vi "GUILoop_plotUpdate_cmds.vi"(0 "reference":refnum<class "OSA.lvclass">, 2 "action data in":T1[](array[typedef]) {"par 4" format="%.2f"; "par 3" format="%.2f"; "par 2" format="%.2f"; "par" format="%.2f"}, 5 "error in (no error)":errorcluster, 6 "action interferogram":cluster{"action":T2, "skip old":bool}[](array[cluster]), 8 "action spectrum":cluster{"action":T2, "skip old":bool}[](array[cluster])) -> (14 "reference out":refnum<class "OSA.lvclass">, 16 "action data out":T1[](array[typedef]) {"par 4" format="%.2f"; "par 3" format="%.2f"; "par 2" format="%.2f"; "par" format="%.2f"}, 19 "error out":errorcluster)   [LabVIEW 2010, in "OSA.lvclass"]
doc: "SubVI to a <B>Thorlabs_OSA_64</B> object.\n\n[GOOP 1.0]"
uses:
  OSA.lvclass
  typeDef/queue_action.ctl
  action_data.ctl
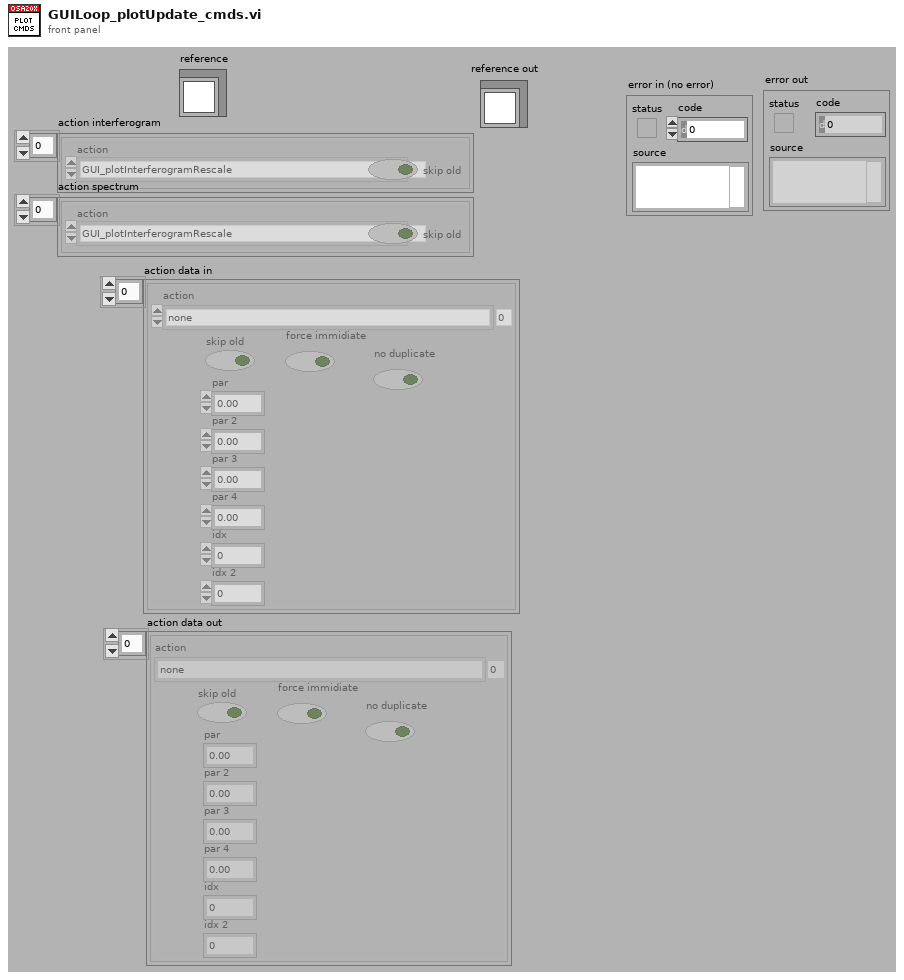
[diagram p1: front panel]
types:
  T1 = typedef "OSA.lvclass/action_data.ctl" = cluster{"action":T2, "skip old":bool, "force immidiate":bool, "par":dbl, "par 2":dbl, "par 3":dbl, "par 4":dbl, "idx":i32, "idx 2":i32, "no duplicate":bool}
  T2 = typedef "OSA.lvclass/queue_action.ctl" = enum16{"none", "stop", "GUI_plotInterferogram", "GUI_plotSpectrum", "GUI_plotInterferogramRescale", "GUI_plotSpectrumRescale", "GUI_plotInterferogramReset", "GUI_plotSpectrumReset", "GUI_plotInterferogramAutoScaleY", "GUI_plotSpectrumAutoScaleY", "GUI_plotInterferogramZoomOut", "GUI_plotSpectrumZoomOut", "GUI_plotInterferogramPane", "GUI_plotSpectrumPane", "GUI_plotInterferogramZoomMouse", "GUI_plotSpectrumZoomMouse", "GUI_plotSpectrumFSRY", "GUI_plotInterferogramFSRY", "GUI_spectrumChannelType", "GUI_channel", "ENVIRONMENT temperature", "ENVIRONMENT pressure", "MODE_resolution set", "MODE_resolution get", "MODE_sensitivity set", "MODE_sensitivity get", "MODE_PDTemperature set", "MODE_PDTemperature get", "REBOOT/RESET firmware", "ACQASYNC_acquireSingleSpectrum", "ACQASYNC_continuous start", "ACQASYNC_continuous stop\n", "ACQASYNC_get last interferogram", "ACQASYNC_get last spectrum", "ACQASYNC_get last waveNr", "ACQOPT_interferogram smoothing set", "ACQOPT_interferogram smoothing get", "ACQOPT_spectrum smoothing set", "ACQOPT_spectrum smoothing get", "ACQOPT_apodisation type set", "ACQOPT_apodisation type get", "ACQOPT_phase correction type set", "ACQOPT_phase correction type get", "ACQOPT_acqIntervall_set", "ACQOPT_acqIntervall_get", "ACQOPT_average spectrum set", "ACQOPT_average spectrum get", "ACQOPT_rolling average set", "ACQOPT_rolling average get", "ACQOPT_zero fill factor set", "ACQOPT_zero fill factor get", "ACQOPT_cycle counting set", "ACQOPT_cycle counting get", "ACQOPT_air measure option set", "ACQOPT_air measure option get", "ACQOPT_gainLevel auto get", "ACQOPT_gainLevel auto set", "ACQOPT_gainLevel get", "ACQOPT_gainLevel set", "ACQOPT_offset set", "ACQOPT_attenuator_auto_set", "ACQOPT_attenuator_set", "ACQOPT_getAll", "INSTRUMENT_PROPERTY_range_WaveNr_min", "INSTRUMENT_PROPERTY_range_WaveNr_max", "INSTRUMENT_PROPERTY_reference_wavelength_cm^-1", "INSTRUMENT_PROPERTY_samplesPerRefPeriod", "INSTRUMENT_PROPERTY_resolution_waveNrPercm", "INSTRUMENT_PROPERTY_availableGainLevels", "INSTRUMENT_PROPERTY_status", "CONVERT", "ANALYSE_POWER", "ANALYSE_PEAKS", "ANALYSE_WAVELENGTH", "ANALYSE_SPECTRUM", "ANALYSE_INTERFEROGRAM", "ANALYSE_COHERENCE_LENGTH", "MATH", "MATH_power", "MATH_peaks", "FILE", "miscellaneous"}
  T3 = typedef "OSA.lvclass/acq_dataType.ctl" = enum16{"none", "interferogram", "spectrum"}
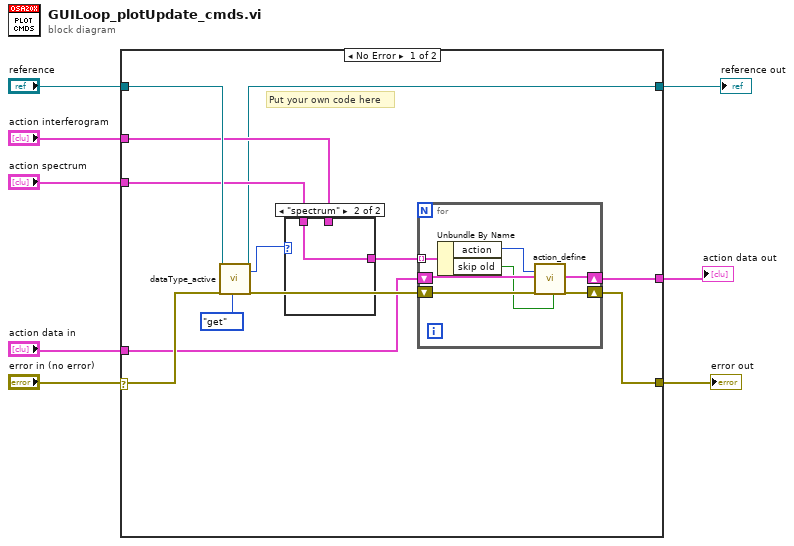
[diagram p0: block diagram]
diagram:
  n1 = case shown="No Error" "error in (no error)" {
    selector: "error in (no error)" -> [w17 w32]
    tunnel: [w10 w32] -> w8
    tunnel: "reference" -> [w18 w31]
    tunnel: [w9 w31] -> w5
    tunnel: "action interferogram" -> [w14 _]
    tunnel: "action spectrum" -> [w15 _]
    tunnel: "action data in" -> [w12 w30]
    tunnel: [w11 w30] -> w1
    frame No Error {
      # "Put your own code here"
      n2 = call "dataType_active.vi"("reference"=w18, "error in (no error)"=w17, "get/set"=enum16{"get", "set"}."get") -> ("duplicate reference"=w9:refnum<class "OSA.lvclass">, "dataType active out"=w20:T3, "error out"=w16:errorcluster)  [unwired: 14 in]
      n3 = case shown="\"spectrum\"" w20 {
        tunnel: w15 -> [_ w29]
        tunnel: w14 -> [w28 _]
        tunnel: [w28 w29] -> w13
        frame "interferogram", Default {
        }
        frame "spectrum" {
        }
      }
      n4 = for {
        shift-right: [w25] -> w11
        shift-left: w12 -> [w24]
        shift-right: [w26] -> w10
        shift-left: w16 -> [w27]
        tunnel: w13 -> [w23] mode=indexing
        n5 = Unbundle By Name(w23) -> ("action"=w22:T2, "skip old"=w21:bool)
        n6 = call "action_define.vi"("action"=w22, "action data"=w24, "error in (no error)"=w27, "skip old"=w21) -> ("action data out"=w25:T1[], "error out"=w26:errorcluster)  [unwired: 14 in]
      }
    }
    frame Error {
      # "Error"
    }
  }
  "error out" <- w8
  "reference out" <- w5
  "action data out" <- w1
